vi "Change Color-space.vi"() -> ()   [LabVIEW 2018]
doc: "Chang Color space: This example is an example of changing the color space, which can change the color space and transform an image from one color representation to another. Color space is a mathematical model that describes colors. Commonly used color spaces include RGB (red, green, blue), HSV (hue, saturation, brightness), HSL (hue, saturation, brightness), YUV, CMYK, etc. Different color spaces have different characteristics."
uses:
  vi.lib/VIRobotics/opencv_yiku/ctls/ColorConversionCodes.ctl
  vi.lib/VIRobotics/opencv_yiku/Mat/Create_Mat_8U.vi
  vi.lib/VIRobotics/opencv_yiku/Mat/Mat_8U/Mat_8U.lvclass
  vi.lib/VIRobotics/opencv_yiku/opencv_yiku.lvlib
panel:
  out "HSV图":picture
  out "灰度图":picture
  out "RGB图":picture
  out "原图":picture
  # "Overview: Demonstrates how to convert images from one color-space to another, like BGR2Gray, BGR2HSV, etc.\nRequirements: Windows.\nInstructions: \n1. Run the VI"
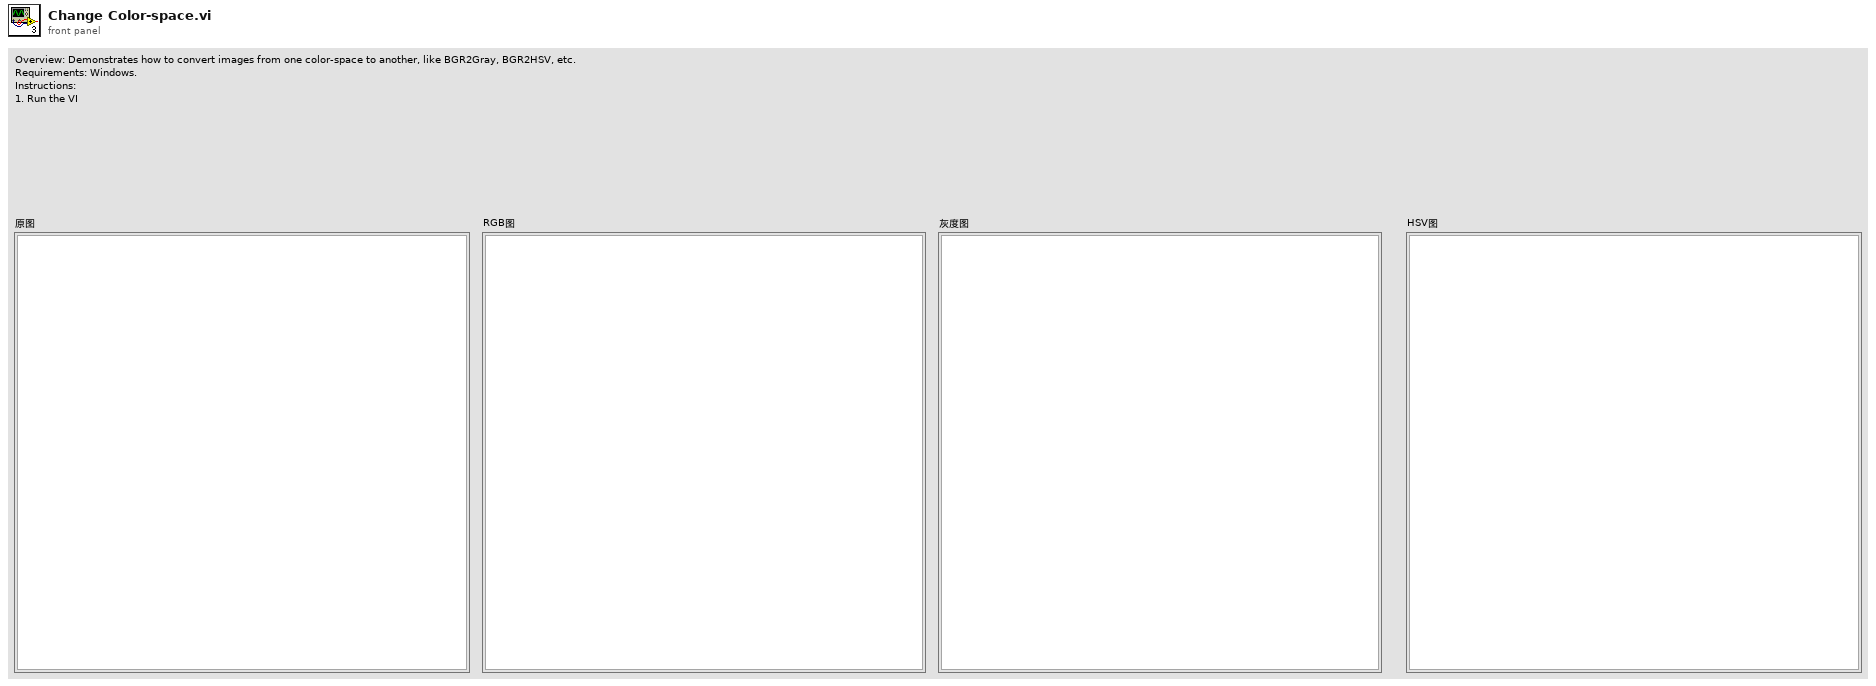
[diagram p1: front panel]
types:
  T1 = typedef "opencv_yiku.lvlib/ColorConversionCodes.ctl" = enum32{"COLOR_BGR2BGRA", "COLOR_BGRA2BGR", "COLOR_BGR2RGBA", "COLOR_RGBA2BGR", "COLOR_BGR2RGB", "COLOR_BGRA2RGBA", "COLOR_BGR2GRAY", "COLOR_RGB2GRAY", "COLOR_GRAY2BGR", "COLOR_GRAY2BGRA", "COLOR_BGRA2GRAY", "COLOR_RGBA2GRAY", "COLOR_BGR2BGR565", "COLOR_RGB2BGR565", "COLOR_BGR5652BGR", "COLOR_BGR5652RGB", "COLOR_BGRA2BGR565", "COLOR_RGBA2BGR565", "COLOR_BGR5652BGRA", "COLOR_BGR5652RGBA", "COLOR_GRAY2BGR565", "COLOR_BGR5652GRAY", "COLOR_BGR2BGR555", "COLOR_RGB2BGR555", "COLOR_BGR5552BGR", "COLOR_BGR5552RGB", "COLOR_BGRA2BGR555", "COLOR_RGBA2BGR555", "COLOR_BGR5552BGRA", "COLOR_BGR5552RGBA", "COLOR_GRAY2BGR555", "COLOR_BGR5552GRAY", "COLOR_BGR2XYZ", "COLOR_RGB2XYZ", "COLOR_XYZ2BGR", "COLOR_XYZ2RGB", "COLOR_BGR2YCrCb", "COLOR_RGB2YCrCb", "COLOR_YCrCb2BGR", "COLOR_YCrCb2RGB", "COLOR_BGR2HSV", "COLOR_RGB2HSV", "42", "43", "COLOR_BGR2Lab", "COLOR_RGB2Lab"}
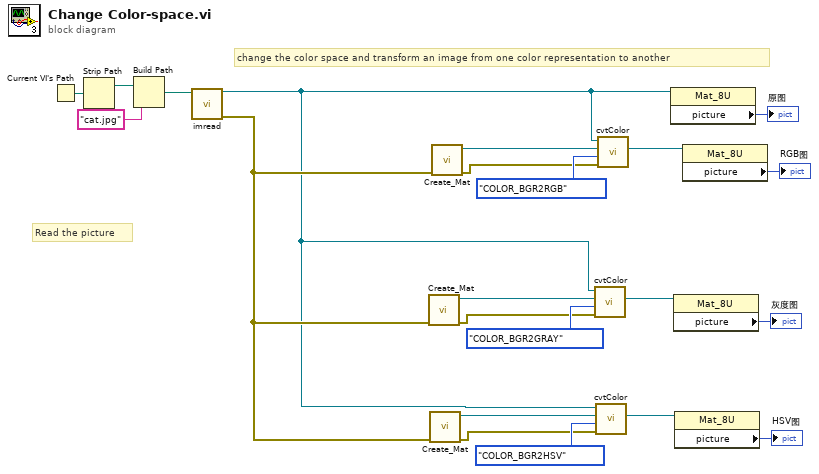
[diagram p0: block diagram]
diagram:
  # "Read the picture"
  # "change the color space and transform an image from one color representation to another"
  n1 = Current VI's Path() -> (path=w20:path)
  n2 = Strip Path(path=w20) -> (stripped path=w22:path)  [unwired: 1 out]
  n3 = Build Path(base path=w22, name or relative path="cat.jpg") -> (appended path=w19:path)
  n4 = call "imread.vi"("path"=w19) -> ("error out"=w2:errorcluster, "Mat out"=w1:refnum<class "Mat_8U.lvclass">)  [unwired: 9 in]
  n5 = call-poly "Create_Mat.vi"("error in (no error)"=w2) -> ("error out"=w13:errorcluster, "Mat_8U_out"=w14:refnum<class "Mat_8U.lvclass">)  [unwired: 9 in]
  n6 = call-poly "Create_Mat.vi"("error in (no error)"=w2) -> ("error out"=w5:errorcluster, "Mat_8U_out"=w6:refnum<class "Mat_8U.lvclass">)  [unwired: 9 in]
  n7 = call-poly "Create_Mat.vi"("error in (no error)"=w2) -> ("error out"=w16:errorcluster, "Mat_8U_out"=w17:refnum<class "Mat_8U.lvclass">)  [unwired: 9 in]
  n8 = call "cvtColor.vi"("error in (no error)"=w13, "dstCn"=ColorConversionCodes."COLOR_BGR2GRAY", "dst"=w14, "src"=w1) -> ("dst out"=w8:refnum<class "Mat_8U.lvclass">)  [unwired: 5 in, 2 out]
  n9 = call "cvtColor.vi"("error in (no error)"=w5, "dstCn"=ColorConversionCodes."COLOR_BGR2HSV", "dst"=w6, "src"=w1) -> ("dst out"=w3:refnum<class "Mat_8U.lvclass">)  [unwired: 5 in, 2 out]
  n10 = call "cvtColor.vi"("error in (no error)"=w16, "dstCn"=ColorConversionCodes."COLOR_BGR2RGB", "dst"=w17, "src"=w1) -> ("dst out"=w10:refnum<class "Mat_8U.lvclass">)  [unwired: 5 in, 2 out]
  n11 = property class="Mat_8U"(reference=w1) -> ("picture"=→"原图":picture)  [unwired: 1 in, 2 out]
  n12 = property class="Mat_8U"(reference=w8) -> ("picture"=→"灰度图":picture)  [unwired: 1 in, 2 out]
  n13 = property class="Mat_8U"(reference=w3) -> ("picture"=→"HSV图":picture)  [unwired: 1 in, 2 out]
  n14 = property class="Mat_8U"(reference=w10) -> ("picture"=→"RGB图":picture)  [unwired: 1 in, 2 out]
